vi "SysLog_Control.vi"(8 "error in (no error)":errorcluster, 11 "Message_Queues":T1) -> (0 "error out":errorcluster)   [LabVIEW 2014]
uses:
  02_Controls/Message_Queues.ctl
  02_Controls/Message_Data_Ctl.ctl
panel:
  out "System Log":string
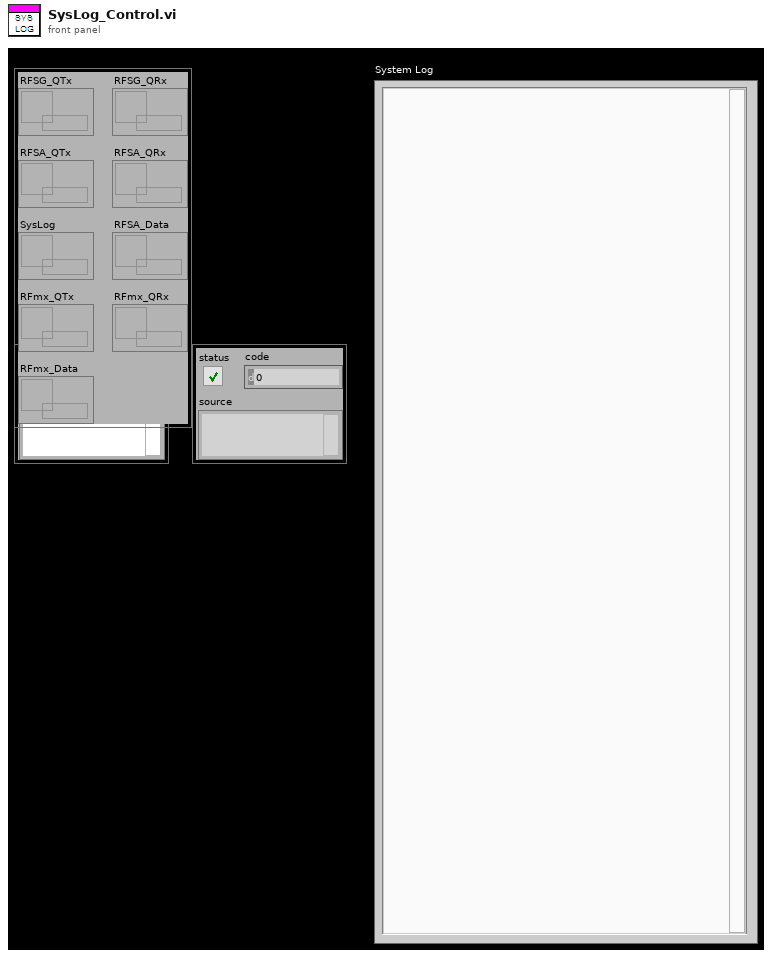
[diagram p1: front panel]
types:
  T1 = typedef "Message_Queues.ctl" = cluster{"RFSG_QTx":refnum<queue>, "RFSG_QRx":refnum<queue>, "RFSA_QTx":refnum<queue>, "RFSA_QRx":refnum<queue>, "SysLog":refnum<queue>, "RFSA_Data":refnum<queue>, "RFmx_QTx":refnum<queue>, "RFmx_QRx":refnum<queue>, "RFmx_Data":refnum<queue>}
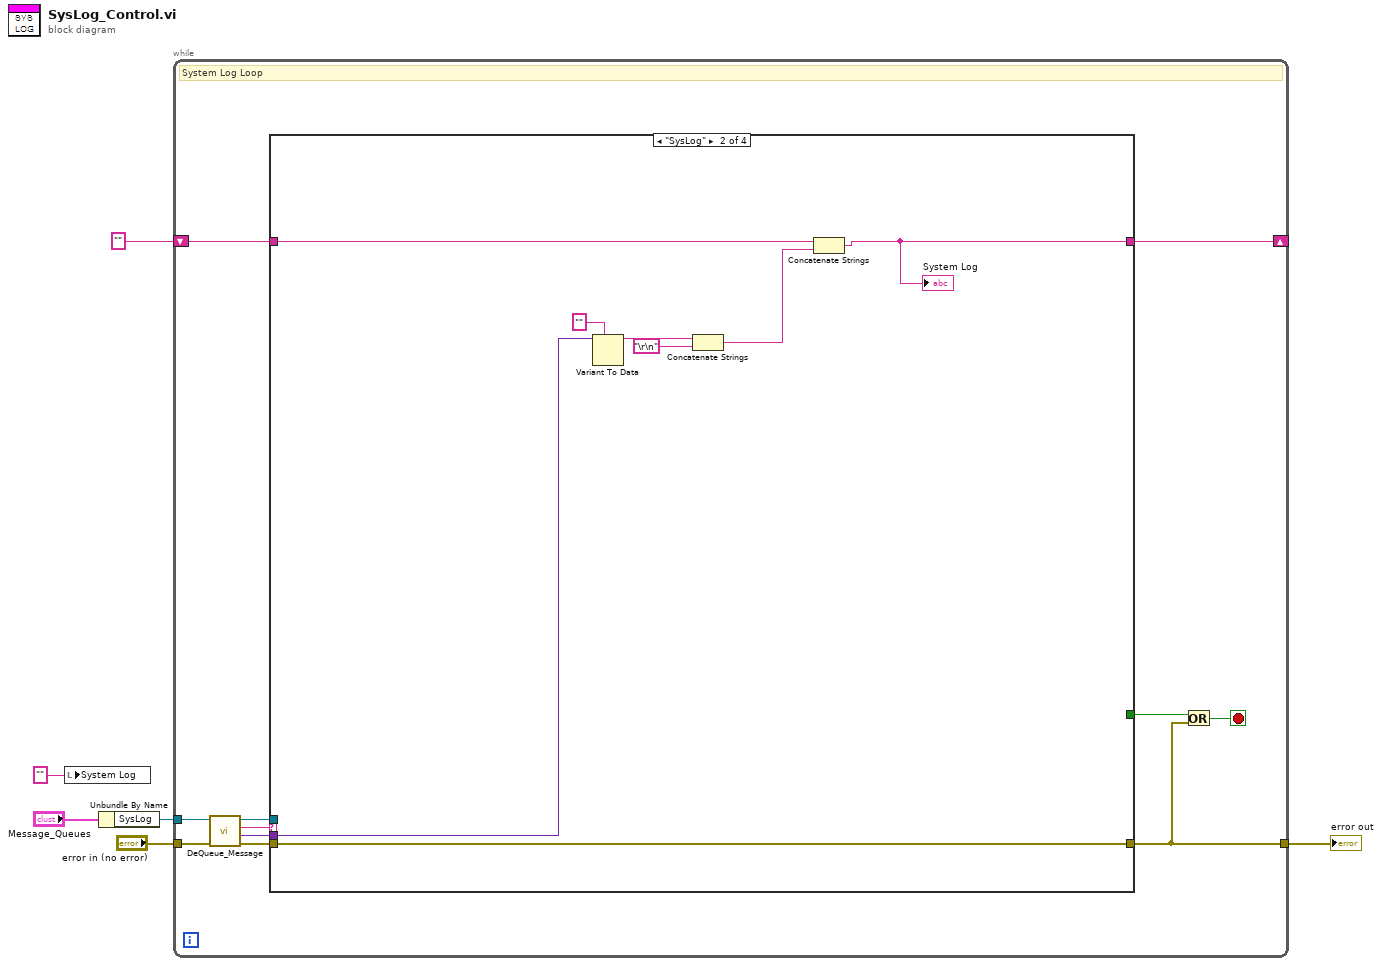
[diagram p0: block diagram]
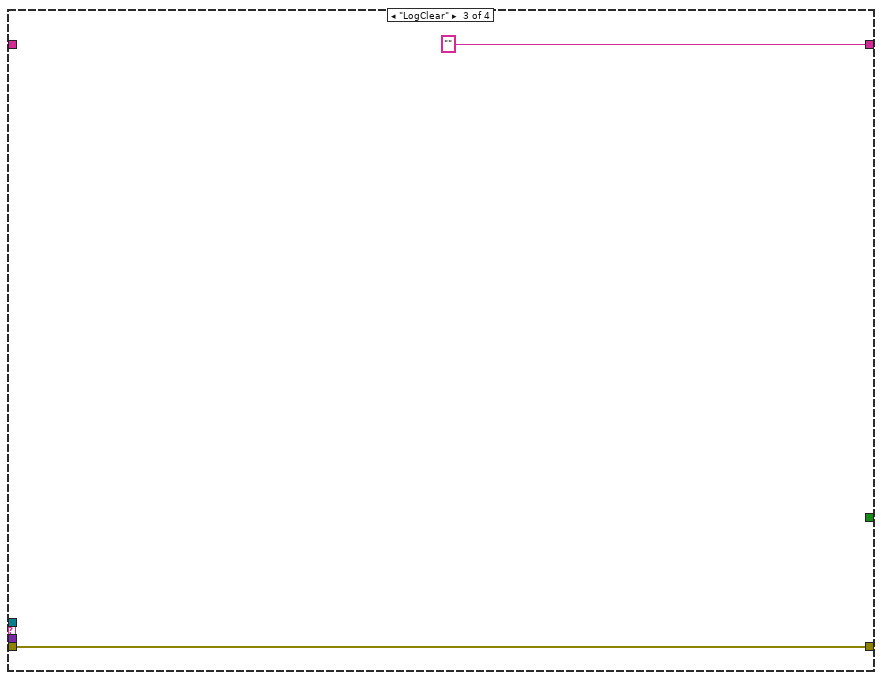
[diagram p3: hidden frame]
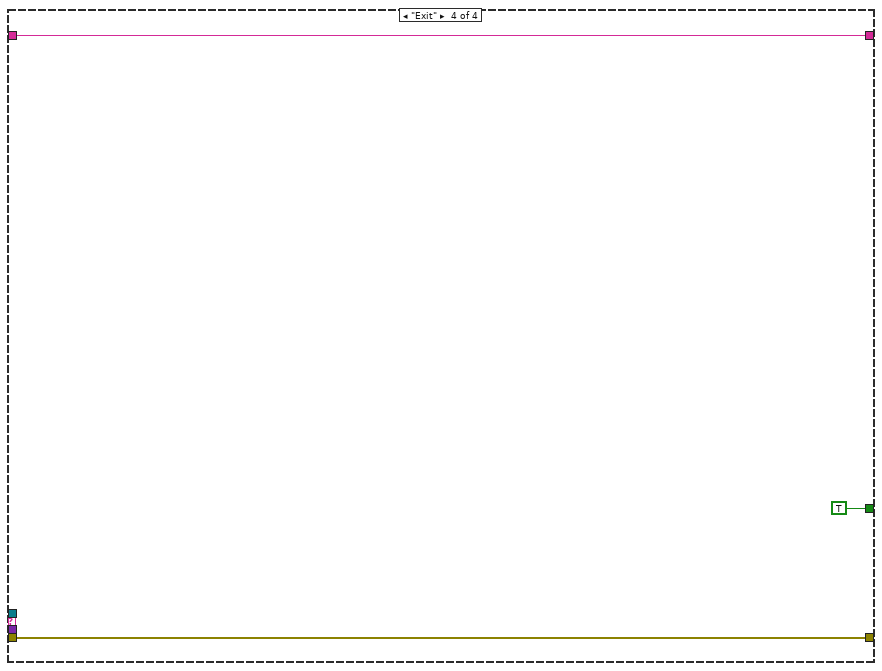
[diagram p4: hidden frame]
diagram:
  n1 = local write "System Log"("" ("System Log")) -> ()
  n2 = Unbundle By Name("Message_Queues") -> ("SysLog"=w4:refnum<queue>)
  n3 = while {
    tunnel: "error in (no error)" -> [w17]
    tunnel: [w7] -> w5
    tunnel: w4 -> [w10]
    shift-right: [w11] -> _
    shift-left: "" -> [w12]
    stop <- w8 stop-if-true
    # "System Log Loop"
    n4 = call "DeQueue_Message.vi"("error in (no error)"=w17, "Message_Queue"=w10) -> ("error out"=w13:errorcluster, "Message Data"=w15:variant, "Message"=w16:string, "Dup_Message_Queue"=w14:refnum<queue>)  [unwired: 6 in]
    n5 = case shown="\"SysLog\"" w16 {
      tunnel: w15 -> [_ w27 _ _]
      tunnel: w14 -> [_ _ _ _]
      tunnel: w13 -> [w19 w21 w28 w31]
      tunnel: [_ _ _ TRUE] -> w9
      tunnel: [w19 w21 w28 w31] -> w7
      tunnel: w12 -> [w18 w25 _ w30]
      tunnel: [w18 w20 "" w30] -> w11
      frame "Wait", Default {
      }
      frame "SysLog" {
        n6 = Variant To Data(type="", Variant=w27) -> (data=w24:string)  [unwired: 1 in, 1 out]
        n7 = Concatenate Strings(w24, "\r\n") -> (w22:string)
        n8 = Concatenate Strings(w25, w22) -> (w20:string)
        "System Log" <- w20
      }
      frame "LogClear" {
      }
      frame "Exit" {
      }
    }
    n9 = Or(x=w9, y=w7) -> (x .or. y?=w8:bool)
  }
  "error out" <- w5
